vi "subVI QCam Get Exposures.vi"(5 "error In":errorcluster, 6 "cameraId In":u32) -> (0 "error out":errorcluster, 1 "qExposure Blue":dbl, 2 "qExposure Red":dbl, 3 "qExposure":dbl, 4 "cameraId out":u32)   [LabVIEW 2012]
doc: "Reads exposure values from camera, return values are in milliseconds."
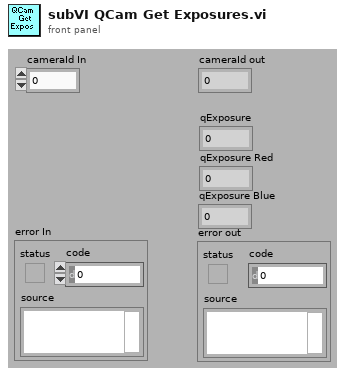
[diagram p1: front panel]
types:
  T1 = enum32{"gain", "offset", "exposure", "binning", "horizontal binning", "vertical binning", "readout speed", "trigger type", "lcd filter", "cooler", "exposure red", "exposure blue", "image format", "roi x", "roi y", "roi width", "roi height", "reserved1", "shutter state", "reserved2", "sync-b out", "reserved3", "intensifier gain", "trigger delay", "camera mode", "normalized gain", "normalized intenifier gain DB", "doPostProcessing", "postProcessGainRed", "postProcessGainGreen", "postProcessGainBlue", "postProcessBayerAlgorithm", "postProcessImageFormat", "fan", "blackout mode", "high sensitivity", "Readout Port", "EM Gain", "open delay", "close delay", "clearing mode"}
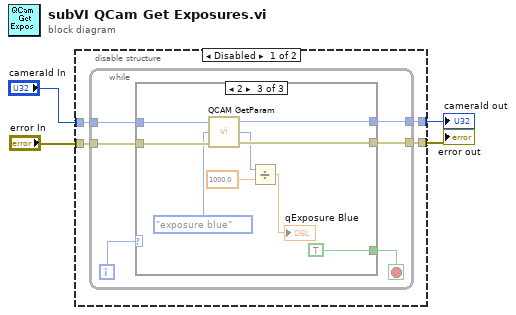
[diagram p0: block diagram]
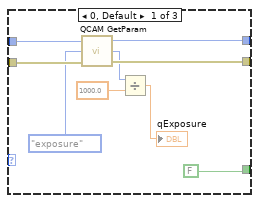
[diagram p2: hidden frame]
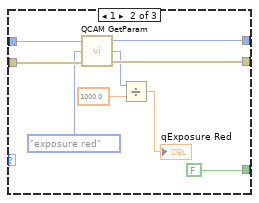
[diagram p3: hidden frame]
diagram:
  n1 = disable-structure shown="Disabled" {
    disable-tunnel: [w8 _] -> w4
    disable-tunnel: [w7 _] -> w3
    disable-tunnel: "error In" -> [w6 _]
    disable-tunnel: "cameraId In" -> [w5 _]
    frame Disabled {
      n2 = while {
        tunnel: w5 -> [w13]
        tunnel: w6 -> [w12]
        tunnel: [w10] -> w7
        tunnel: [w9] -> w8
        i -> [w14]
        stop <- w11 stop-if-true
        n3 = case shown="2" w14 {
          tunnel: w13 -> [w23 w32 w41]
          tunnel: w12 -> [w22 w31 w40]
          tunnel: [FALSE FALSE TRUE] -> w11
          tunnel: [w18 w28 w36] -> w10
          tunnel: [w19 w27 w37] -> w9
          frame 0, Default {
            n4 = call "QCAM GetParam.vi"("cameraId in"=w23, "parameter key"=T1."exposure", "error in (no error)"=w22) -> ("cameraId out"=w19:u32, "value out"=w15:u32, "error out"=w18:errorcluster)  [unwired: 2 out]
            n5 = Divide(x=w15, y=1000.0) -> (x/y=→"qExposure":dbl)
          }
          frame 1 {
            n6 = call "QCAM GetParam.vi"("cameraId in"=w32, "parameter key"=T1."exposure red", "error in (no error)"=w31) -> ("cameraId out"=w27:u32, "value out"=w24:u32, "error out"=w28:errorcluster)  [unwired: 2 out]
            n7 = Divide(x=w24, y=1000.0) -> (x/y=→"qExposure Red":dbl)
          }
          frame 2 {
            n8 = call "QCAM GetParam.vi"("cameraId in"=w41, "parameter key"=T1."exposure blue", "error in (no error)"=w40) -> ("cameraId out"=w37:u32, "value out"=w33:u32, "error out"=w36:errorcluster)  [unwired: 2 out]
            n9 = Divide(x=w33, y=1000.0) -> (x/y=→"qExposure Blue":dbl)
          }
        }
      }
    }
    frame Enabled {
    }
  }
  "cameraId out" <- w4
  "error out" <- w3
